vi "--decorator.vi"(4 "Sender":refnum<class "Sender.lvclass">, 7 "Actor in":refnum<class "Actor.lvclass">, 10 "Pump State":bool) -> (0 "Error out":errorcluster, 5 "Actor out":refnum<class "Actor.lvclass">)   [LabVIEW 2025, in "Update Pump State Msg.lvlib"]
uses:
  Update Pump State Msg.lvlib
  <vilib>/Nathan Davis/jettl/jettl/jettl/Sender/Sender/Sender.lvclass
  <vilib>/Nathan Davis/jettl/jettl/jettl/Actor/Actor/Actor.lvclass
  Update Pump State Msg/Update Pump State Msg.lvclass
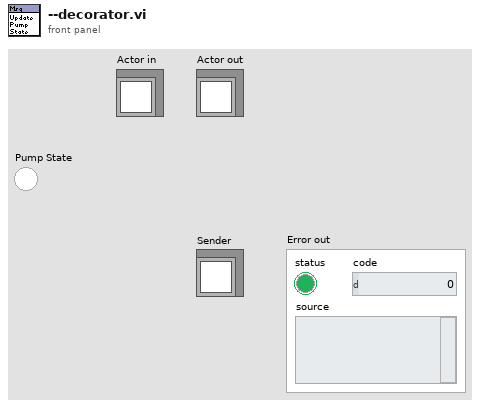
[diagram p1: front panel]
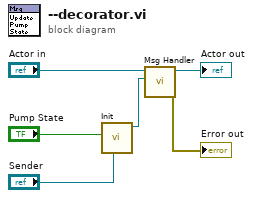
[diagram p0: block diagram]
diagram:
  n1 = call "Init.vi"("Sender"="Sender", "Pump State"="Pump State") -> ("Update Pump State Msg out"=w1:refnum<class "Update Pump State Msg.lvclass">)  [unwired: 9 in]
  n2 = call-dynamic "Msg Handler.vi"("Msg"=w1, "Actor in"="Actor in") -> ("Error out"=→"Error out":errorcluster, "Actor out"=→"Actor out":refnum<class "Actor.lvclass">)  [unwired: 8 in]
